vi "Low Pass Filtering.vi"() -> ()   [LabVIEW 2014]
uses:
  <vilib>/Analysis/3filter.llb/Filter Passband Type.ctl
  <vilib>/FPGAPlugInAG/sbRIO-9636/niLvFpga_Open_sbRIO-9636.vi
  <vilib>/rvi/interface/common/dynamic/niFpgaDynamicAddResources.vi
  <vilib>/Utility/error.llb/Error Cluster From Error Code.vi
  <vilib>/rvi/errors/niLvFpgaAdjustHostInterfaceError.vi
  <vilib>/rvi/interface/common/niFpgaWaitOnOcc.vi
  <vilib>/FPGAPlugInAG/Dynamic/niLvFpga_Run_Dynamic.vi
  <vilib>/RVI Host/nirviSupport.llb/nirviErrorClusterFromErrorCode.vi
  <vilib>/Analysis/3filter.llb/Butterworth Filter (DBL).vi
  <vilib>/FPGAPlugInAG/Dynamic/niLvFpga_Reset_Dynamic.vi
  <vilib>/FPGAPlugInAG/Dynamic/niLvFpga_Abort_Dynamic.vi
  <vilib>/rvi/interface/nirviOpenFPGA/nirviOpenFPGA.xnode
  FPGA Bitfiles/LaserDistanceSen_FPGATarget_EstrazioneFondo_lh4CFmKzsjs.lvbitx
  FPGA Target/Support VIs/Estrazione Fondo.vi
  <vilib>/rvi/interface/nirviReadWriteControl/nirviReadWriteControl.xnode
  <vilib>/rvi/interface/nirviMethod/nirviMethod.xnode
  <vilib>/FPGAPlugInAG/Dynamic/niLvFpga_ConfigureFifo_Dynamic.vi
  <vilib>/rvi/errors/niLvFpgaMergeErrorWithErrorCode.vi
  <vilib>/FPGAPlugInAG/Dynamic/niLvFpga_StartFifo_Dynamic.vi
  <vilib>/Analysis/NI_AALBase.lvlib
  <vilib>/FPGAPlugInAG/Dynamic/niLvFpga_AcknowledgeIrq_Dynamic.vi
  <vilib>/rvi/interface/nirviMethod/StockFPGA_InlinedMethodWaitForSingleIRQ.vi
  <vilib>/FPGAPlugInAG/Dynamic/niLvFpga_WaitOnIrq_Dynamic.vi
  <vilib>/FPGAPlugInAG/Dynamic/niLvFpga_WriteFifo_Dynamic.vi
  <vilib>/FPGAPlugInAG/Dynamic/niLvFpga_ReadFifo_Dynamic.vi
  NiFpgaLv.dll
  <vilib>/rvi/interface/Simulation/niFpgaSimulationCallBeginRW.vi
panel:
  out "Numero di misure mediate":dbl
  in  "Low cutoff frequency":dbl=20000.0 format="%#_13g"
  out "Subtracted signal Low Pass Filter":dbl[](graph)
  in  "N (potenza del due => 2^N)":i32=8
  out "Low Pass Filter Result":dbl[](graph)
  out "Complete Signal Mean":dbl[](graph)
  # "LOW PASS FILTER"
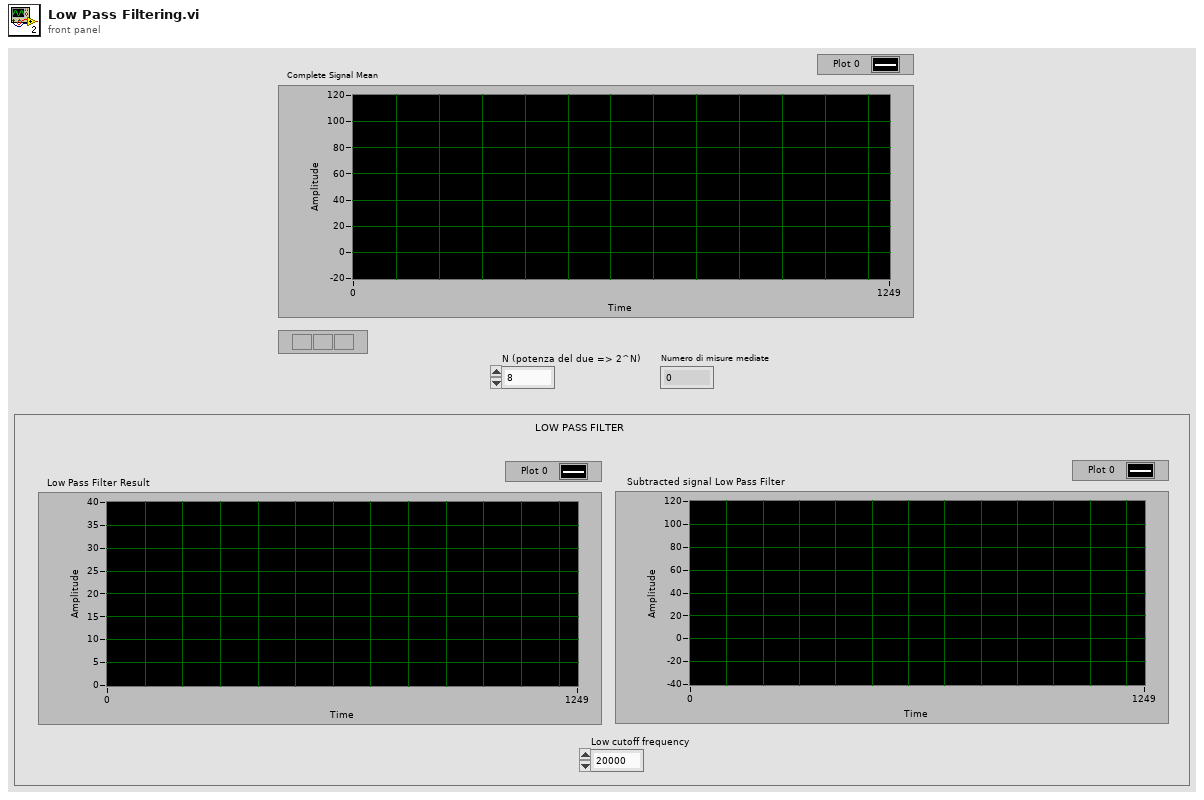
[diagram p1: front panel]
types:
  T1 = typedef "NI_AALBase.lvlib/Filter Passband Type.ctl" = enum32{"Lowpass", "Highpass", "Bandpass", "Bandstop"}
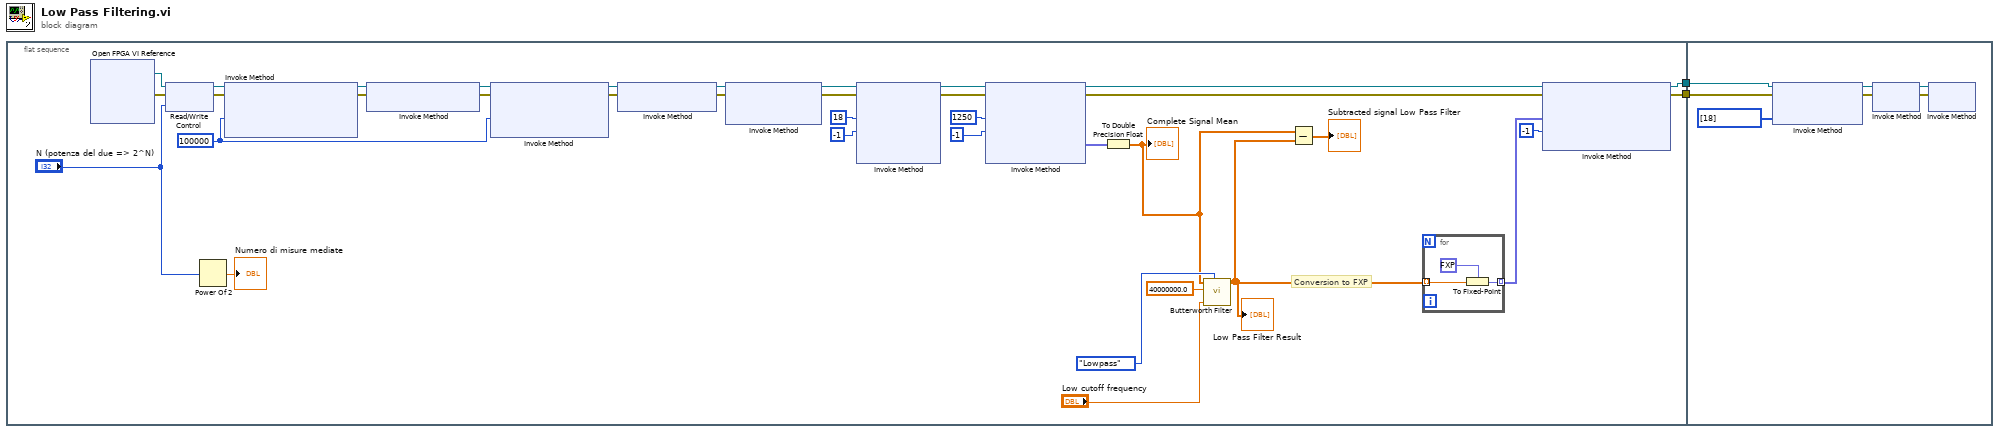
[diagram p0: block diagram]
diagram:
  n1 = flat-sequence {
    tunnel: [w27] -> w2
    tunnel: [w26] -> w1
    tunnel: w2 -> [w48]
    tunnel: w1 -> [w47]
    frame #0 {
      w25 = u32 100000 ("Requested Depth")
      # "Conversion to FXP"
      n2 = xnode "Open FPGA VI Reference"() -> ("FPGA VI Reference Out"=w12:refnum<k20>, "error out"=w14:errorcluster)  [unwired: 2 in]
      n3 = xnode "Read/Write Control"("FPGA VI Reference In"=w12, "error in"=w14, "N-Mean"="N (potenza del due => 2^N)") -> ("FPGA VI Reference Out"=w11:refnum<k20>, "error out"=w13:errorcluster)
      n4 = Power Of 2(x="N (potenza del due => 2^N)") -> (2^x=→"Numero di misure mediate":dbl)
      n5 = xnode "Invoke Method"("FPGA VI Reference In"=w11, "error in"=w13, "Requested Depth"=w25) -> ("FPGA VI Reference Out"=w24:refnum<k20>, "error out"=w23:errorcluster)  [unwired: 1 out]
      n6 = xnode "Invoke Method"("FPGA VI Reference In"=w24, "error in"=w23) -> ("FPGA VI Reference Out"=w22:refnum<k20>, "error out"=w21:errorcluster)
      n7 = xnode "Invoke Method"("FPGA VI Reference In"=w22, "error in"=w21, "Requested Depth"=w25) -> ("FPGA VI Reference Out"=w38:refnum<k20>, "error out"=w37:errorcluster)  [unwired: 1 out]
      n8 = xnode "Invoke Method"("FPGA VI Reference In"=w38, "error in"=w37) -> ("FPGA VI Reference Out"=w18:refnum<k20>, "error out"=w17:errorcluster)
      n9 = xnode "Invoke Method"("FPGA VI Reference In"=w18, "error in"=w17) -> ("FPGA VI Reference Out"=w16:refnum<k20>, "error out"=w15:errorcluster)  [unwired: 1 in]
      n10 = xnode "Invoke Method"("FPGA VI Reference In"=w16, "error in"=w15, "IRQ Number(s)"=18, "Timeout (ms)"=-1) -> ("FPGA VI Reference Out"=w7:refnum<k20>, "error out"=w6:errorcluster)  [unwired: 2 out]
      n11 = xnode "Invoke Method"("FPGA VI Reference In"=w7, "error in"=w6, "Number of Elements"=u32 1250, "Timeout (ms)"=-1) -> ("FPGA VI Reference Out"=w31:refnum<k20>, "error out"=w30:errorcluster, "Data"=w10:fxp<+/-,12,12>[])  [unwired: 1 out]
      n12 = To Double Precision Float(number=w10) -> (double precision float=w8:dbl[])
      "Complete Signal Mean" <- w8
      n13 = call-poly <vilib>:"Butterworth Filter.vi"("filter type"=Filter_Passband_Type."Lowpass", "low cutoff freq: fl"="Low cutoff frequency", "sampling freq: fs"=40000000.0, "X"=w8) -> ("Filtered X"=w3:dbl[])  [unwired: 4 in, 1 out]
      "Low Pass Filter Result" <- w3
      n14 = Subtract(x=w8, y=w3) -> (x-y=→"Subtracted signal Low Pass Filter":dbl[])
      n15 = for {
        tunnel: w3 -> [w41] mode=indexing
        tunnel: [w39] -> w29 mode=indexing
        n16 = To Fixed-Point(fixed-point type=fxp<+/-,12,12> 0.0, number=w41) -> (fixed-point=w39:fxp<+/-,12,12>)
      }
      n17 = xnode "Invoke Method"("FPGA VI Reference In"=w31, "error in"=w30, "Data"=w29, "Timeout (ms)"=-1) -> ("FPGA VI Reference Out"=w27:refnum<k20>, "error out"=w26:errorcluster)  [unwired: 1 out]
    }
    frame #1 {
      n18 = xnode "Invoke Method"("FPGA VI Reference In"=w48, "error in"=w47, "IRQ Number(s)"=i32[] [18]) -> ("FPGA VI Reference Out"=w45:refnum<k20>, "error out"=w44:errorcluster)
      n19 = xnode "Invoke Method"("FPGA VI Reference In"=w45, "error in"=w44) -> ("FPGA VI Reference Out"=w43:refnum<k20>, "error out"=w42:errorcluster)
      n20 = xnode "Invoke Method"("FPGA VI Reference In"=w43, "error in"=w42) -> ()  [unwired: 2 out]
    }
  }
